vi "Get Data.vi"(8 "error in":errorcluster, 11 "tCRD in":refnum<class "Aircraft OPCCRD.lvclass">) -> (0 "error out":errorcluster, 3 "tCRD out":refnum<class "Aircraft OPCCRD.lvclass">)   [LabVIEW 2015, in "Aircraft OPCCRD.lvclass"]
doc: "Retrieve the data from the given cards. Set the <B>goodData</B> flag to True and log any errors that will be handled down the line. If there is an error associated with the collection of the data, the <B>goodData</B> flag will be set to false when the logged errors are handled.\nThe ringdown traces recorded in the <B>HF AI</B> task are divided up into a m x n matrix where:\n * m = YAG pulse rate\n * n = YAG duty cycle * HF AI Sampling Rate / YAG Pulse Rate"
uses:
  Aircraft OPCCRD.lvclass
  Reusable/Instrument/state.ctl
  Reusable/CRDS/Main/Read Data.vi
  Reusable/Data/Write measTime.vi
  Reusable/CRDS/Main/Write Data.vi
  Reusable/CRDS/Main/Write goodData.vi
  Reusable/CRDS/Data/Main/CRDS Data.lvclass
  Reusable/Instrument/Instrument.lvclass
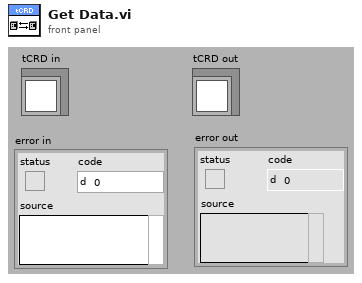
[diagram p1: front panel]
types:
  T1 = typedef "Instrument.lvclass/state.ctl" = enum8{"Configure", "Acquire", "Wait", "Quit", "Handle Error", "NOOP"}
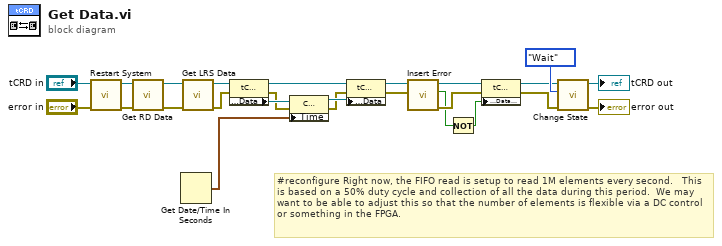
[diagram p0: block diagram]
diagram:
  # "#reconfigure Right now, the FIFO read is setup to read 1M elements every second.   This is based on a 50% duty cycle and collection of all the data during this period.  We may want to be able to adjust this so that the number of elements is flexible via a DC control or something in the FPGA."
  n1 = call "Restart System.vi"("error in"="error in", "tCRD in"="tCRD in") -> ("error out"=w16:errorcluster, "tCRD out"=w13:refnum<class "Aircraft OPCCRD.lvclass">)  [unwired: 8 in]
  n2 = call "Get RD Data.vi"("error in"=w16, "tCRD in"=w13) -> ("error out"=w9:errorcluster, "tCRD out"=w12:refnum<class "Aircraft OPCCRD.lvclass">)  [unwired: 8 in]
  n3 = Get Date/Time In Seconds() -> (seconds since 1Jan1904=w8:timestamp)
  n4 = call "Get LRS Data.vi"("error in"=w9, "tCRD in"=w12) -> ("error out"=w10:errorcluster, "tCRD out"=w11:refnum<class "Aircraft OPCCRD.lvclass">)  [unwired: 8 in]
  n5 = property class="tCRD"(reference=w11, error in=w10) -> (reference out=w5:refnum<class "Aircraft OPCCRD.lvclass">, error out=w6:errorcluster, "Data Access:Data"=w7:refnum<class "CRDS Data.lvclass">)
  n6 = property class="CRDS"(reference=w7, error in=w6, "Time"=w8) -> (reference out=w2:refnum<class "CRDS Data.lvclass">, error out=w1:errorcluster)
  n7 = property class="tCRD"(reference=w5, error in=w1, "Data Access:Data"=w2) -> (reference out=w4:refnum<class "Aircraft OPCCRD.lvclass">, error out=w3:errorcluster)
  n8 = call "Insert Error.vi"("err"=w3, "Instrument in"=w4) -> ("error out"=w21:errorcluster, "error?"=w18:bool, "Instrument out"=w22:refnum<class "Aircraft OPCCRD.lvclass">)  [unwired: 7 in]
  n9 = Not(x=w18) -> (.not. x?=w17:bool)
  n10 = property class="tCRD"(reference=w22, error in=w21, "Data Access:Data Ready?"=w17) -> (reference out=w20:refnum<class "Aircraft OPCCRD.lvclass">, error out=w19:errorcluster)
  n11 = call "Change State.vi"("error in"=w19, "instr state"=state."Wait", "Instrument in"=w20) -> ("error out"=→"error out":errorcluster, "Instrument out"=→"tCRD out":refnum<class "Aircraft OPCCRD.lvclass">)  [unwired: 7 in]
